vi "Ex 1 starging Func Gen.vi"() -> ()   [LabVIEW 2025]
uses:
  <vilib>/sound2/lvsound2.llb/Sound Data Format.ctl
  <vilib>/measure/maspectr.llb/FFT Power Spectrum and PSD for 1 Chan.vi
  <vilib>/sound2/lvsound2.llb/Sound Output Write (DBL Single).vi
  <vilib>/sound2/lvsound2.llb/Sound Output Write (DBL).vi
  <vilib>/measure/NI_MAPro.lvlib
  <vilib>/measure/NI_MABase.lvlib
panel:
  out "Waveform Graph":waveform(dbl)(graph)
  out "Spectrum":cluster{"f0":dbl, "df":dbl, "magnitude":dbl[]}(graph)
  out "Signal":waveform(dbl)(graph)
  in  "length pts":dbl=30000.0
  in  "dt":dbl=0.0001
  in  "Freq Stop":dbl=500.0
  in  "Freq Start":dbl=100.0
  in  "Amp":dbl=1.0
  in  "Amplitude":dbl=2.0
  in  "Frequency":dbl=10.0
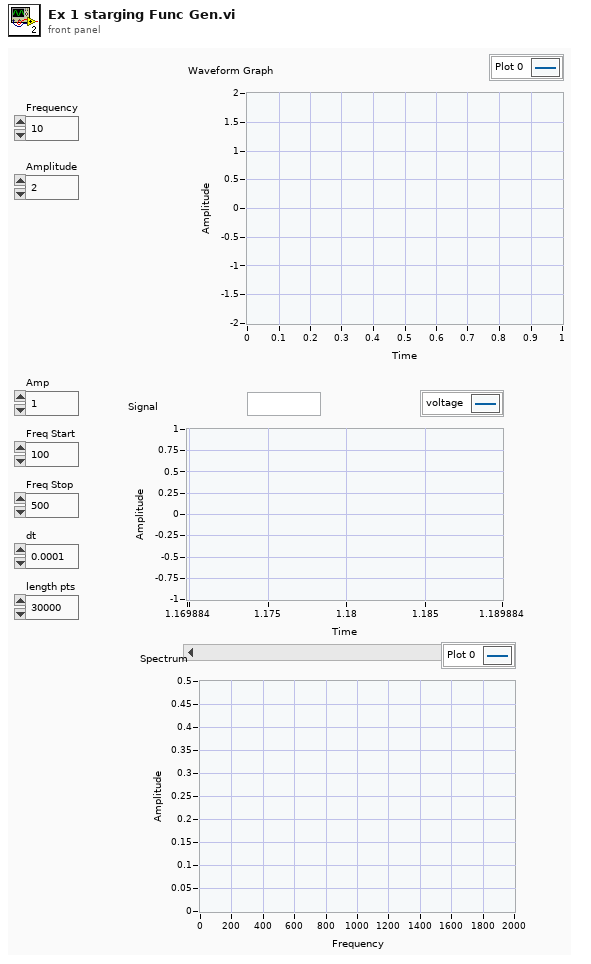
[diagram p1: front panel]
types:
  T1 = typedef "Sound Data Format.ctl" = cluster{"sample rate (S/s)":dbl, "number of channels":i32, "bits per sample":i32}
  T2 = enum16{"Sine Wave", "Triangle Wave", "Square Wave", "Sawtooth Wave"}
  T3 = typedef "Sound Output Task ID.ctl" = u32
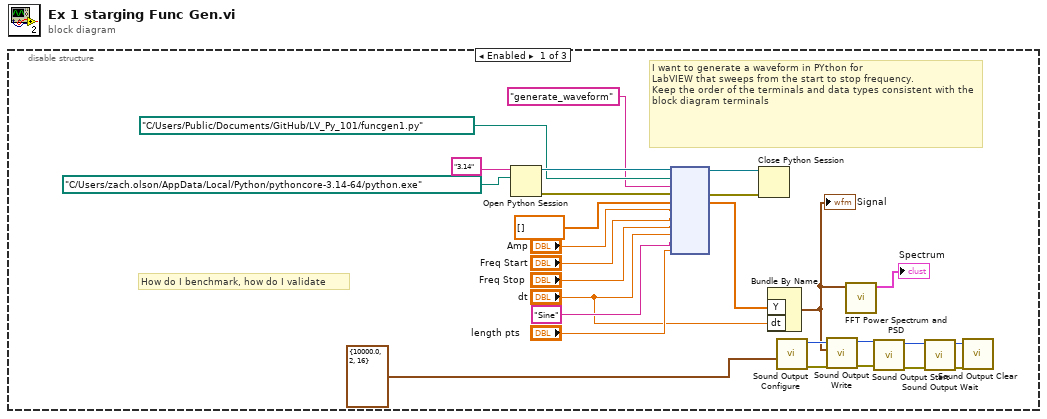
[diagram p0: block diagram]
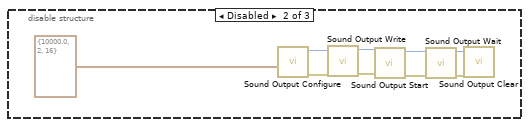
[diagram p2: hidden frame]
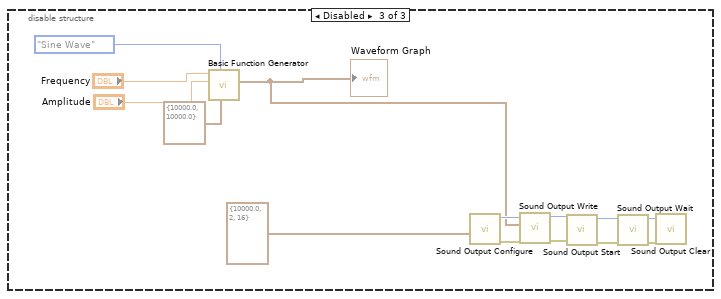
[diagram p3: hidden frame]
diagram:
  n1 = disable-structure shown="Enabled" {
    frame Enabled {
      # "I want to generate a waveform in PYthon for \nLabVIEW that sweeps from the start to stop frequency.\nKeep the order of the terminals and data types consistent with the block diagram terminals"
      # "How do I benchmark, how do I validate"
      n2 = Open Python Session(python version="3.14" ("Python version"), python path=path "C:/Users/zach.olson/AppData/Local/Python/pythoncore-3.14-64/python.exe" ("Python path")) -> (session out=w25:refnum<k35>, error out=w24:errorcluster)  [unwired: 1 in]
      n3 = node(w25, path "C:/Users/Public/Documents/GitHub/LV_Py_101/funcgen1.py" ("module path"), "generate_waveform" ("function name"), w24, dbl[] [], "Amp", "Freq Start", "Freq Stop", "dt", "Sine", "length pts") -> (w23:refnum<k35>, w22:errorcluster, w5:dbl[])  [unwired: 6 in, 2 out]
      n4 = Close Python Session(session in=w23, error in=w22) -> ()  [unwired: 1 out]
      n5 = Bundle By Name("Y"=w5, "dt"="dt") -> (w2:waveform(dbl))  [unwired: 1 in]
      "Signal" <- w2
      n6 = call <vilib>:"Sound Output Configure.vi"("sound format"=T1 {"sample rate (S/s)"=10000.0, "number of channels"=2, "bits per sample"=16}) -> ("error out"=w6:errorcluster, "task ID"=w7:T3)  [unwired: 9 in]
      n7 = call-poly <vilib>:"Sound Output Write.vi"("error in (no error)"=w6, "data"=w2, "task ID"=w7) -> ("error out"=w8:errorcluster, "task ID out"=w9:T3)  [unwired: 7 in]
      n8 = call-poly <vilib>:"FFT Power Spectrum and PSD.vi"("time signal"=w2) -> ("Power Spectrum / PSD"=→"Spectrum":cluster{"f0":dbl, "df":dbl, "magnitude":dbl[]})  [unwired: 7 in, 3 out]
      n9 = call <vilib>:"Sound Output Start.vi"("error in (no error)"=w8, "task ID"=w9) -> ("error out"=w10:errorcluster, "task ID out"=w11:T3)  [unwired: 8 in]
      n10 = call <vilib>:"Sound Output Wait.vi"("error in (no error)"=w10, "task ID"=w11) -> ("error out"=w13:errorcluster, "task ID out"=w12:T3)  [unwired: 8 in]
      n11 = call <vilib>:"Sound Output Clear.vi"("error in (no error)"=w13, "task ID"=w12) -> ()  [unwired: 9 in, 1 out]
    }
    frame Disabled {
      n12 = call <vilib>:"Sound Output Configure.vi"("sound format"=T1 {"sample rate (S/s)"=10000.0, "number of channels"=2, "bits per sample"=16}) -> ("error out"=w29:errorcluster, "task ID"=w30:T3)  [unwired: 9 in]
      n13 = call-poly <vilib>:"Sound Output Write.vi"("error in (no error)"=w29, "task ID"=w30) -> ("error out"=w31:errorcluster, "task ID out"=w32:T3)  [unwired: 8 in]
      n14 = call <vilib>:"Sound Output Start.vi"("error in (no error)"=w31, "task ID"=w32) -> ("error out"=w33:errorcluster, "task ID out"=w34:T3)  [unwired: 8 in]
      n15 = call <vilib>:"Sound Output Wait.vi"("error in (no error)"=w33, "task ID"=w34) -> ("error out"=w36:errorcluster, "task ID out"=w35:T3)  [unwired: 8 in]
      n16 = call <vilib>:"Sound Output Clear.vi"("error in (no error)"=w36, "task ID"=w35) -> ()  [unwired: 9 in, 1 out]
    }
    frame Disabled {
      n17 = call <vilib>:"Basic Function Generator.vi"("sampling info"=cluster{"Fs":dbl, "#s":dbl} {"Fs"=10000.0, "#s"=10000.0}, "signal type"=T2."Sine Wave", "amplitude"="Amplitude", "frequency"="Frequency") -> ("signal out"=w37:waveform(dbl))  [unwired: 5 in, 2 out]
      "Waveform Graph" <- w37
      n18 = call <vilib>:"Sound Output Configure.vi"("sound format"=T1 {"sample rate (S/s)"=10000.0, "number of channels"=2, "bits per sample"=16}) -> ("error out"=w40:errorcluster, "task ID"=w41:T3)  [unwired: 9 in]
      n19 = call-poly <vilib>:"Sound Output Write.vi"("error in (no error)"=w40, "data"=w37, "task ID"=w41) -> ("error out"=w42:errorcluster, "task ID out"=w43:T3)  [unwired: 7 in]
      n20 = call <vilib>:"Sound Output Start.vi"("error in (no error)"=w42, "task ID"=w43) -> ("error out"=w44:errorcluster, "task ID out"=w45:T3)  [unwired: 8 in]
      n21 = call <vilib>:"Sound Output Wait.vi"("error in (no error)"=w44, "task ID"=w45) -> ("error out"=w47:errorcluster, "task ID out"=w46:T3)  [unwired: 8 in]
      n22 = call <vilib>:"Sound Output Clear.vi"("error in (no error)"=w47, "task ID"=w46) -> ()  [unwired: 9 in, 1 out]
    }
  }
